vi "frequency_response.vi"() -> ()   [LabVIEW 2012]
uses:
  Trace controls.ctl
  probe_point.ctl
  injection_point.ctl
  pose_selector.ctl
  pose_source.ctl
  pose_relative_to.ctl
  <vilib>/Platform/TimedLoop/XDataNode/timing_clust.ctl
  <vilib>/Platform/TimedLoop/XDataNode/nitl_modes.ctl
  <vilib>/Platform/TimedLoop/XDataNode/wakeup.ctl
  <vilib>/Utility/error.llb/DialogType.ctl
  <vilib>/Utility/file.llb/Write To Spreadsheet File (string).vi
  initialization/micron_globals.vi
  <vilib>/Platform/TimedLoop/XDataNode/XDataNode.xnode
  <vilib>/Platform/TimedLoop/XDataNode/XDNodeRunTimeDep.lvlib
  <vilib>/Analysis/NI_AALPro.lvlib
  <vilib>/gmath/NI_Gmath.lvlib
panel:
  in  "Pose response":T1[](array[typedef])
  in  "Use Output Enable":bool=TRUE
  out "Report":string[][](table)
  in  "Report file":path=path "c:/test/freq_reponse.csv"
  in  "Save report":bool
  in  "Store":T4(radio)=enum."Radio Selection 7"
  in  "Graph?":bool[](array[boolean])=[TRUE, TRUE, TRUE, TRUE, TRUE, TRUE, FALSE]
  in  "Name":string[](array[string])
  in  "Delay":sgl=0.0031 format="%#_3p"
  out "Responses":waveform(sgl)[](graph)
  out "Reference":waveform(sgl)[](graph)
  in  "Reference signal":T5[](array[typedef])=[{"+ stim"=TRUE, "Relative"=FALSE, "Scale"=enum."1X", "Probe point"=enum."Output 0", "XYZ selector"={"Boolean"=TRUE, "Boolean 2"=FALSE, "Boolean 3"=FALSE}, "To tip"=FALSE}, {"+ stim"=FALSE, "Relative"=FALSE, "Scale"=enum."1X", "Probe point"=enum."Position (tip)", "XYZ selector"={"Boolean"=FALSE, "Boolean 2"=FALSE, "Boolean 3"=FALSE}, "To tip"=FALSE}, {"+ stim"=FALSE, "Relative"=FALSE, "Scale"=enum."1X", "Probe point"=enum."Position (tip)", "XYZ selector"={"Boolean"=FALSE, "Boolean 2"=FALSE, "Boolean 3"=FALSE}, "To tip"=FALSE}, {"+ stim"=FALSE, "Relative"=FALSE, "Scale"=enum."1X", "Probe point"=enum."Position (tip)", "XYZ selector"={"Boolean"=FALSE, "Boolean 2"=FALSE, "Boolean 3"=FALSE}, "To tip"=FALSE}]
  out "Driven axis":i32
  in  "Scanning":bool
  in  "Scan":bool
  in  "Stimulus":T8={"Injection point"=enum."Output", "Closed loop"=TRUE, "Tip -> world"=FALSE, "Amplitude"=10.0, "Type"=enum."Arbitrary", "Phase"=0.0, "Frequency"=0.0, "Length"=0.0} {"Length" min=0.0 max=100.0 step=100.0 format="%#_4p"; "Frequency" min=0.0 step=100.0 format="%#_4g"; "Phase" min=-180.0 max=360.0 step=100.0 format="%#.2f"; "Amplitude" format="%#_3p"}
  in  "Scan axes":bool[](array[boolean])=[TRUE, TRUE, TRUE, TRUE, TRUE, TRUE]
  in  "Max off-axis":bool=TRUE
  in  "Integrator scaling":bool=TRUE
  in  "Frequency range":cluster{"Min":dbl, "Max":dbl}={"Min"=10.0, "Max"=250.0} {"Max" format="%#_3p"; "Min" format="%#_3p"}
  in  "N points":u32=30
  in  "Window":T9(ring)
  in  "Restart Averaging":bool
  in  "Unwrap phase":bool
  in  "Averaging Parameters":T10={"averaging mode"=0, "weighting mode"=1, "number of averages"=10} {"averaging mode" items=["No averaging", "Vector averaging", "RMS averaging", "Peak hold"]; "weighting mode" items=["Linear", "Exponential"]}
  in  "Phase offset":sgl=90.0
  out "Status":string
  out "Phase":T11(graph)
  out "Amplitude":cluster{"X":dbl[], "Y":dbl[]}[](graph)
  in  "Response signals":T5[](array[typedef])=[{"+ stim"=FALSE, "Relative"=FALSE, "Scale"=enum."1X", "Probe point"=enum."Link pos 0", "XYZ selector"={"Boolean"=TRUE, "Boolean 2"=TRUE, "Boolean 3"=TRUE}, "To tip"=FALSE}, {"+ stim"=FALSE, "Relative"=FALSE, "Scale"=enum."1X", "Probe point"=enum."Link pos 1", "XYZ selector"={"Boolean"=TRUE, "Boolean 2"=TRUE, "Boolean 3"=TRUE}, "To tip"=FALSE}, {"+ stim"=FALSE, "Relative"=FALSE, "Scale"=enum."1X", "Probe point"=enum."Position (tip)", "XYZ selector"={"Boolean"=FALSE, "Boolean 2"=FALSE, "Boolean 3"=FALSE}, "To tip"=FALSE}, {"+ stim"=FALSE, "Relative"=FALSE, "Scale"=enum."1X", "Probe point"=enum."Position (tip)", "XYZ selector"={"Boolean"=FALSE, "Boolean 2"=FALSE, "Boolean 3"=FALSE}, "To tip"=FALSE}]
  # "Result buffers"
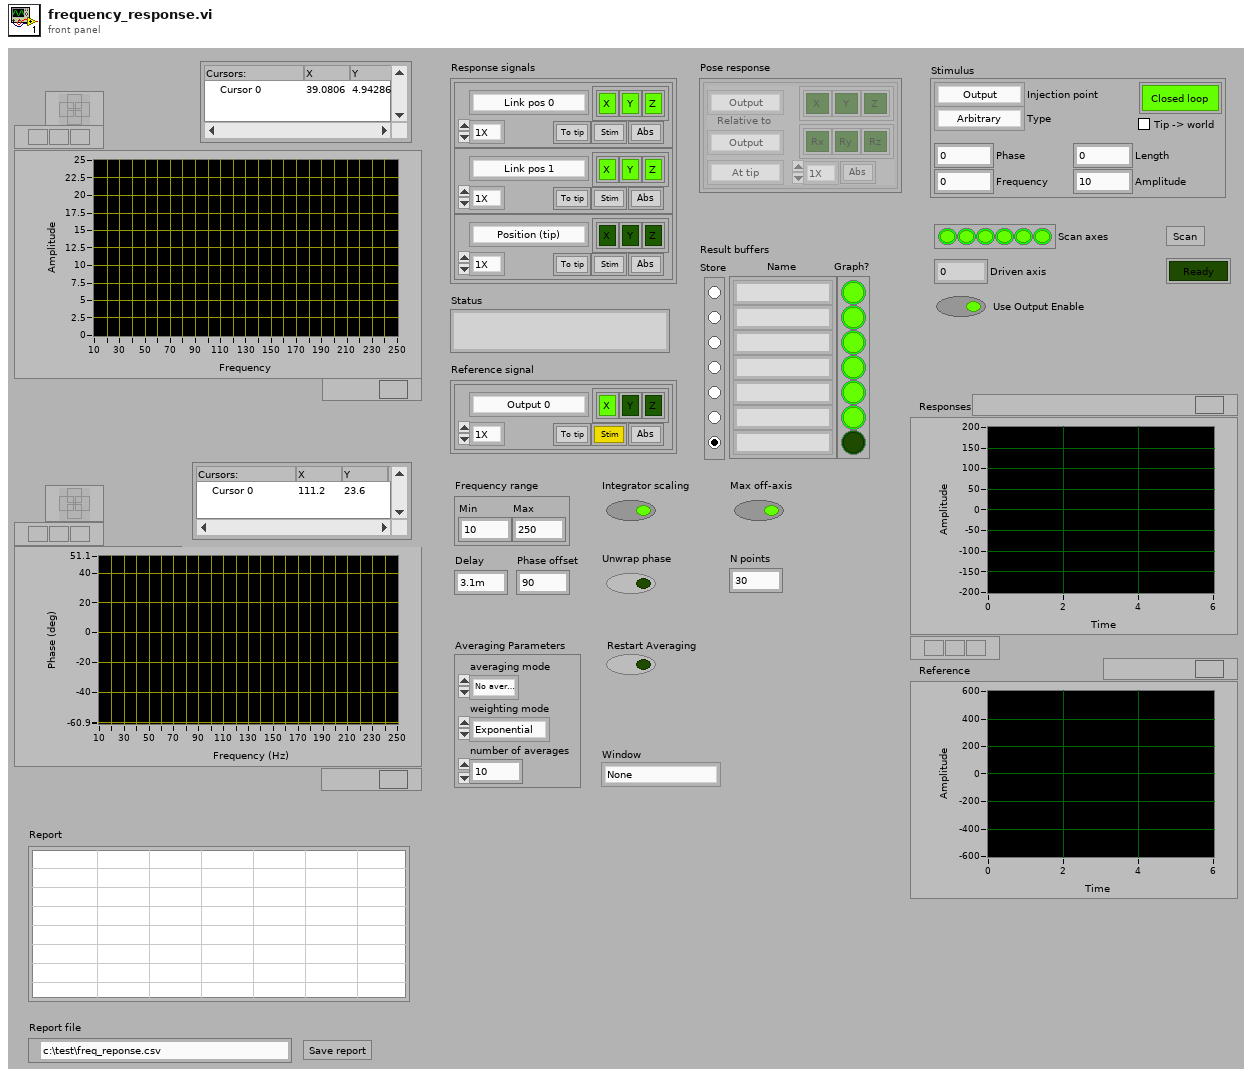
[diagram p1: front panel]
types:
  T1 = typedef "pose_selector.ctl" = cluster{"Scale":enum16{"1X", "10X", "100X", "1KX", "10KX"}, "Source":T2, "XYZ selector":cluster{"Boolean":bool, "Boolean 2":bool, "Boolean 3":bool}, "RPY selector":cluster{"Boolean":bool, "Boolean 2":bool, "Boolean 3":bool}, "Relative to":T3, "Relative":bool, "Translate":enum16{"At tip", "At RCM", "At KC", "At origin"}}
  T2 = typedef "pose_source.ctl" = enum16{"Output", "Handle", "Handle KF", "Goal", "Absolute"}
  T3 = typedef "pose_relative_to.ctl" = enum16{"Output", "Handle", "Handle KF", "Goal", "Absolute", "Trace start"}
  T4 = enum32{"Radio Selection 1", "Radio Selection 2", "Radio Selection 3", "Radio Selection 4", "Radio Selection 5", "Radio Selection 6", "Radio Selection 7"}
  T5 = typedef "Trace controls.ctl" = cluster{"+ stim":bool, "Relative":bool, "Scale":enum16{"1X", "10X", "100X", "1KX", "10KX"}, "Probe point":T6, "XYZ selector":cluster{"Boolean":bool, "Boolean 2":bool, "Boolean 3":bool}, "To tip":bool}
  T6 = typedef "probe_point.ctl" = enum16{"Position (tip)", "Position (RCM)", "Null pos (tip)", "Null pos (RCM)", "V limiter (tip)", "V Limiter (RCM)", "Goal (tip)", "Goal (RCM)", "Link pos 0", "Link pos 1", "KF link pos 0", "KF link pos 1", "Link rate 0", "Link rate 1", "Link residue 0", "Link residue 1", "Link goal 0", "Link goal 1", "Rate limit 0", "Rate limit 1", "Link error 0", "Link error 1", "Controller 0", "Controller 1", "Output 0", "Output 1", "Drive 0", "Drive 1", "Stimulus 0", "Stimulus 1", "Trace data 0", "Trace data 1", "Analog data 0", "Analog data 1", "Status flags", "Light 0", "Light 1", "Light 2", "Light 3", "Light 4", "Light 5", "Goal origin", "Goal rotation 0", "Goal rotation 1", "Goal rotation 2", "Output origin", "Output rotation 0", "Output rotation 1", "Output rotation 2", "Handle origin", "Handle rotation 0", "Handle rotation 1", "Handle rotation 2", "Handle position", "Handle velocity", "Handle acceleration", "Handle angles", "Handle angle rates", "Handle pos residue", "Handle angle residue", "Trace length"}
  T7 = typedef "injection_point.ctl" = enum16{"Total pose", "V limiter", "Goal ", "Link position", "KF link position", "Inverse kin", "Link goal", "Link error", "Controller", "Output", "Drive", "Light"}
  T8 = cluster{"Injection point":T7, "Closed loop":bool, "Tip -> world":bool, "Amplitude":sgl, "Type":enum16{"Off", "Step", "Sine", "Triangle", "Arbitrary"}, "Phase":dbl, "Frequency":dbl, "Length":dbl}
  T9 = enum16{"None ", "Hanning", "Hamming", "Blackman-Harris", "Exact Blackman", "Blackman", "Flat Top", "4 Term B-Harris ", "7 Term B-Harris", "Low Sidelobe"}
  T10 = cluster{"averaging mode":u16, "weighting mode":u16, "number of averages":u32}
  T11 = cluster{"X out":dbl[], "Unwrapped Phase":dbl[]}[]
  T12 = typedef "XDNodeRunTimeDep.lvlib/timing_clust.ctl" = cluster{"Expected End [f-1]":u64, "Actual End [f-1]":u64, "Finished Late? [f-1]":bool, "Expected End [i-1]":u64, "Actual End [i-1]":u64, "Finished Late? [i-1]":bool, "Expected Start [i]":u64, "Actual Start [i]":u64, "Expected Start [f]":u64, "Actual Start [f]":u64, "Source Name":string, "Structure Name":string, "Period":i64, "Deadline":i64, "Offset":i64, "Start":i64, "Priority":i32, "Timeout":i32, "Mode":T13, "Wakeup Reason":T14, "Error":errorcluster, "Source Type":string, "Secondary Source Type":string, "Global End Time":u64, "Global Start Time":u64, "Frame Duration":u64, "Iteration Duration":u64, "Assigned CPU":i32, "I/O Scan Engine Mode":u32}
  T13 = typedef "XDNodeRunTimeDep.lvlib/nitl_modes.ctl" = enum32{"No Change", "Process missed periods, maintain original phase", "Discard missed periods, maintain original phase", "Process missed periods, ignore original phase", "Discard missed periods, ignore original phase"}
  T14 = typedef "XDNodeRunTimeDep.lvlib/wakeup.ctl" = enum32{"Normal", "Aborted", "Asynchronous wakeup", "Timing source error", "Timed loop error", "Timeout"}
  T15 = cluster{"Averaging Parameters":cluster{"averaging mode":u16, "weighting mode":u16, "number of averages":u32}, "Window":enum16{"None ", "Hanning", "Hamming", "Blackman-Harris", "Exact Blackman", "Blackman", "Flat Top", "4 Term B-Harris ", "7 Term B-Harris", "Low Sidelobe"}, "Reference signal":T5[]}
  T16 = cluster{"Phase offset":sgl, "Unwrap phase ":bool, "N points":u32, "Integrator scaling":bool, "Frequency range":cluster{"Min":dbl, "Max":dbl}, "Max off-axis":bool, "Graph?":bool[], "Name":string[], "Delay":sgl}
  T17 = enum8{"Enabled", "Disabled", "Disabled and Grayed Out"}
  T18 = typedef "DialogType.ctl" = u16
  T19 = enum16{"Off", "Step", "Sine", "Triangle", "Arbitrary"}
  T20 = typedef "Micron params.ctl" = cluster{"Stimulus":T21, "Goal Filter A":T22, "Mode controls":T23, "Manipulator type":enum16{"Current piezo", "Voltage piezo"}, "Manipulator calibration":T24, "Network":T26, "Goal Filter B":T22, "Cancellation":T27, "Transition time":sgl, "Estimation":T29}
  T21 = typedef "stimulus.ctl" = cluster{"Type":enum16{"Off", "Step", "Sine", "Triangle", "Arbitrary"}, "Phase":dbl, "Amplitude":sgl[], "Injection point":T7, "Closed loop":bool, "Offset":sgl[], "Tip -> world":bool, "Frequency":dbl, "Length":dbl}
  T22 = typedef "goal_loop_parms.ctl" = cluster{"Speedup max":sgl, "Speedup thresh":sgl, "Speedup nonlin":sgl, "Filters":cluster{"Lower Fc":sgl, "Lower Q":sgl, "Scale factor":sgl, "Upper Fc":sgl, "Upper Q":sgl, "V limit":sgl, "V limit range":sgl}[]}
  T23 = typedef "mode_conrols.ctl" = cluster{"Hold":bool, "Cancellation":bool, "Goal filter":bool, "Trigger":bool}
  T24 = typedef "manipulator_cal.ctl" = cluster{"Tool offsets":sgl[][], "Tip light calibration":T25, "Handle light calibration":T25, "Base pivots":sgl[][], "Output pivots":sgl[][], "Length center":sgl, "Workspace height":sgl[], "Workspace diameter":sgl[], "Linearization":sgl[][], "Stack travel":sgl, "Saturation pos":sgl, "Inverse filters":cluster{"filter structure":enum32{"IIR 2nd Order", "IIR 4th Order"}, "Reverse Coefficients":dbl[], "Forward Coefficients":dbl[]}[]}
  T25 = typedef "probe_calibration.ctl" = sgl[][]
  T26 = typedef "network_params.ctl" = cluster{"Remote Host":string, "Send Status":bool, "Send Port":u16, "Recv Commands":bool, "Recv Port":u16}
  T27 = typedef "sq_control_params.ctl" = cluster{"KP":T28, "KI":sgl, "KD":T28, "Max vel":sgl, "Max acc":sgl, "Int error limit":sgl, "RCM gain":sgl, "Bypass":bool, "Degraded gain":sgl}
  T28 = typedef "decoupled_gain.ctl" = cluster{"XY":sgl, "Rxy":sgl, "Z":sgl, "Rz":sgl}
  T29 = typedef "estimation_controls.ctl" = cluster{"Link":cluster{"Measure noise":dbl[], "Process noise":dbl[], "Alt process noise":dbl[], "Alt turnoff cycles":i32, "Innovation limit":dbl[], "Residue threshold":dbl, "Enable":bool}, "Handle":cluster{"Measure noise":dbl[], "Process noise":dbl[], "State limits":dbl[], "Innovation limit":dbl[], "Prediction Lookahead":sgl, "Enable":bool}}
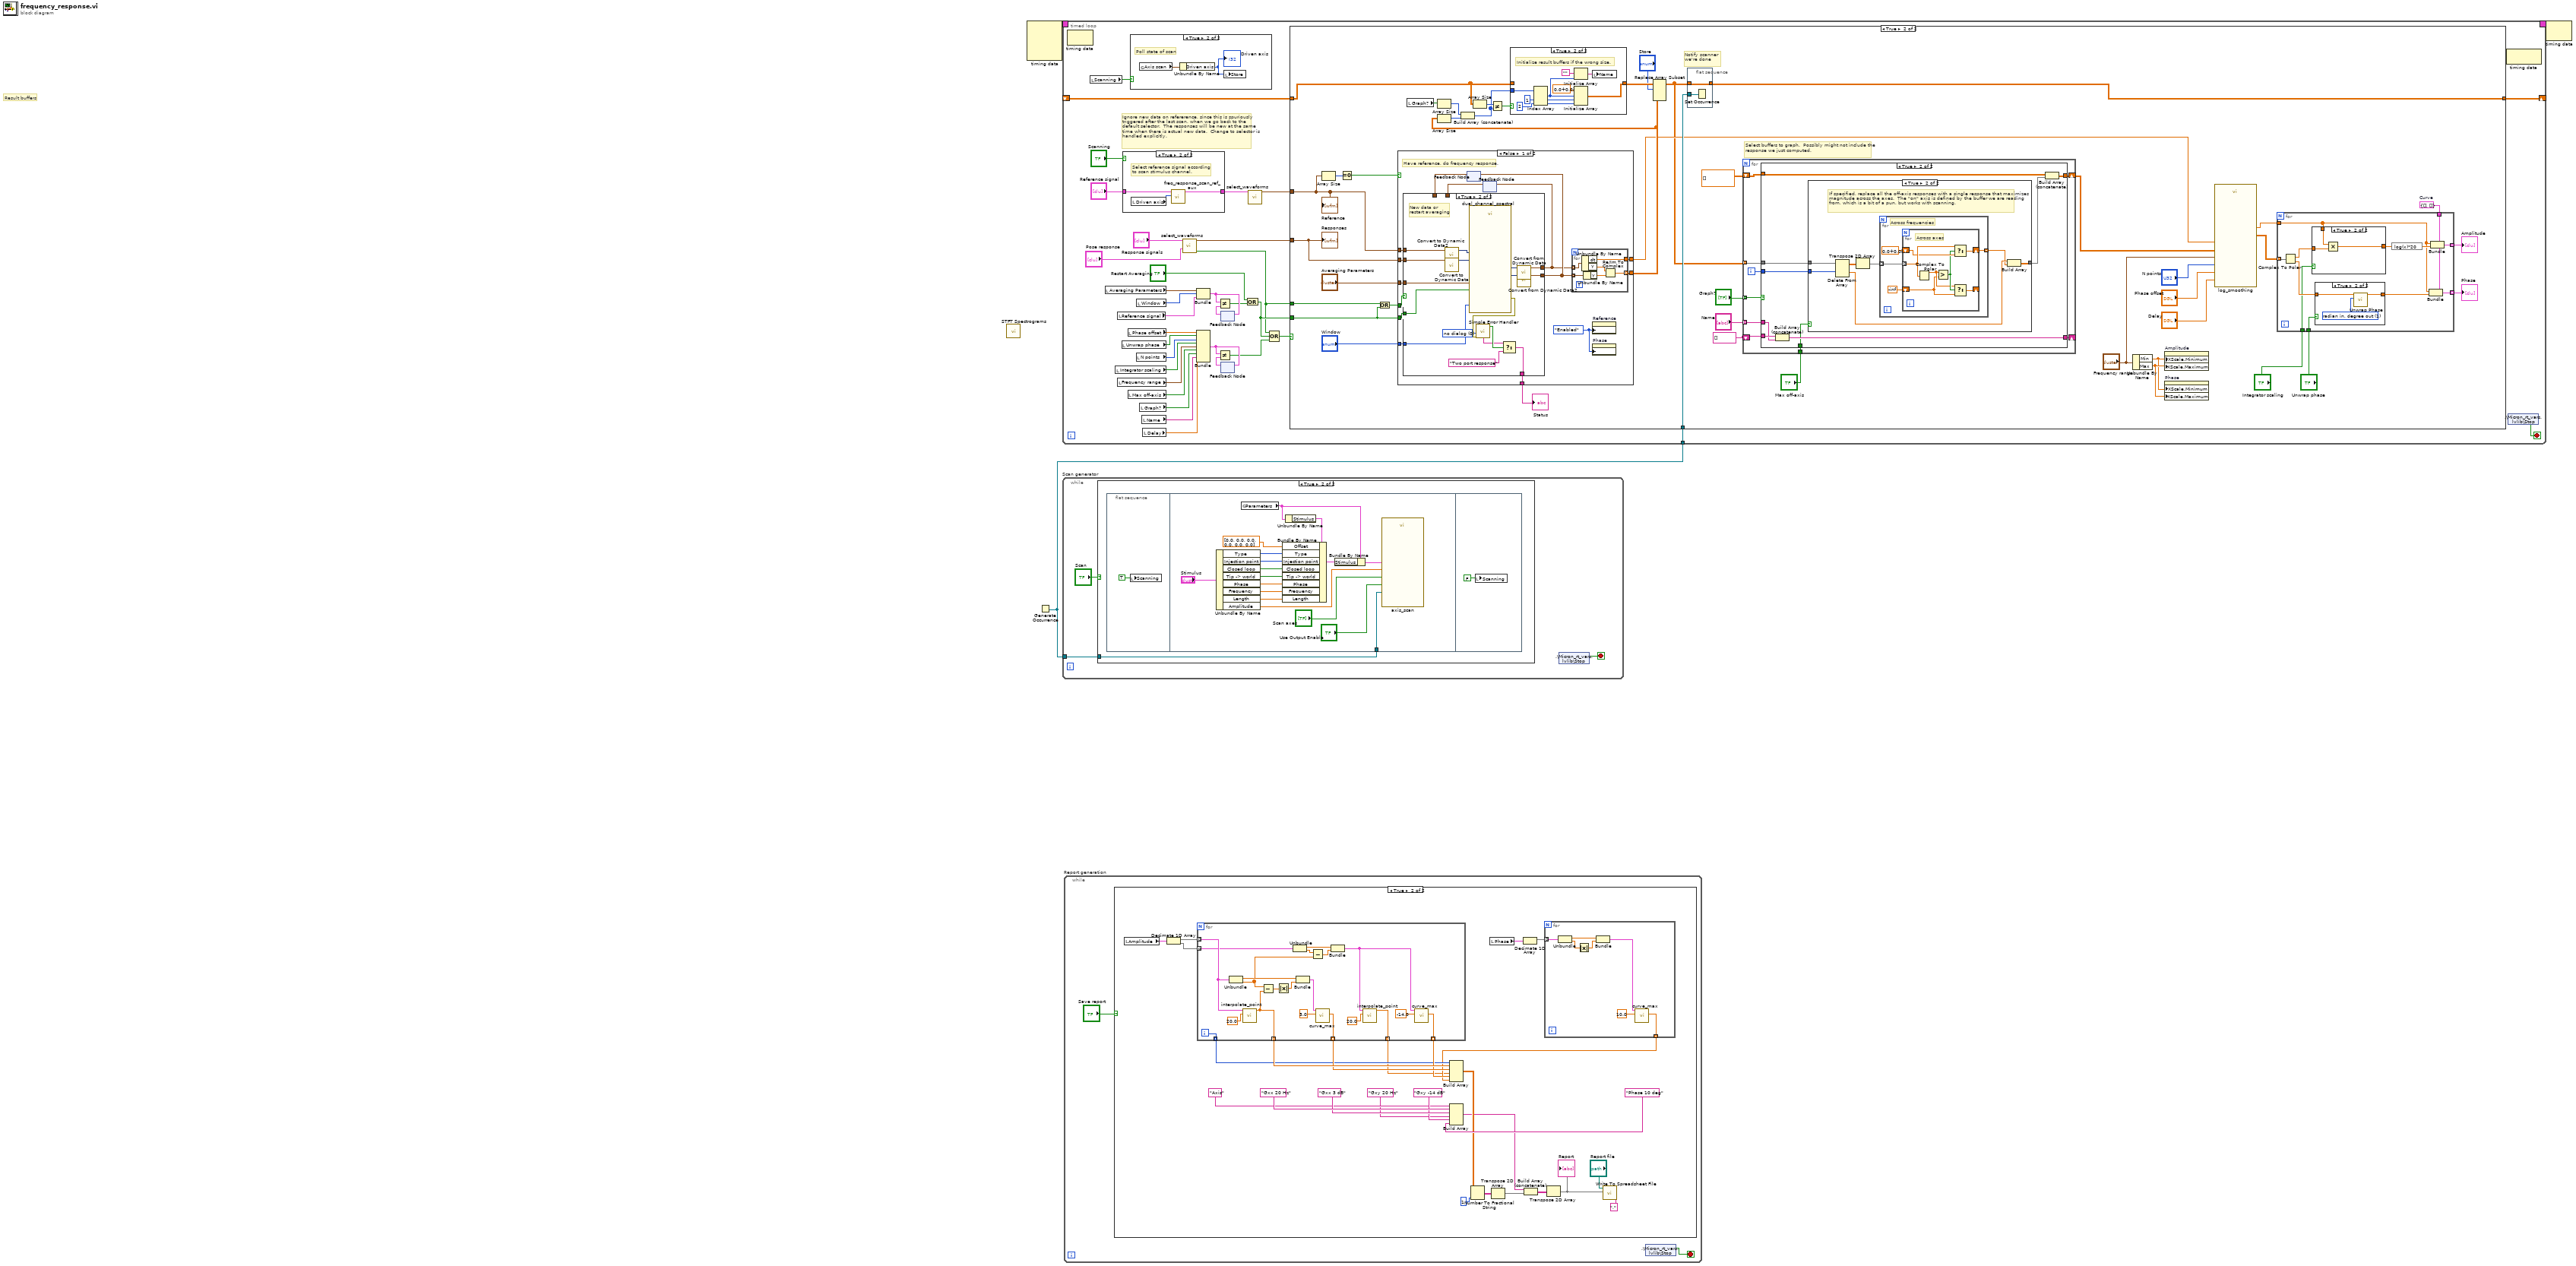
[diagram p0: block diagram]
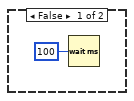
[diagram p2: hidden frame]
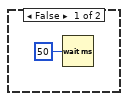
[diagram p3: hidden frame]
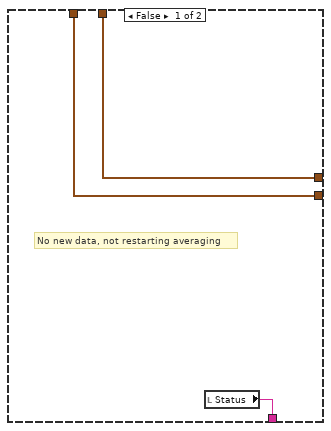
[diagram p7: hidden frame]
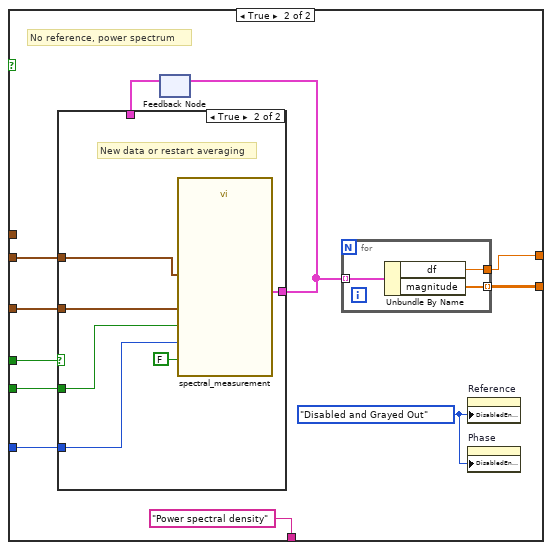
[diagram p8: hidden frame]
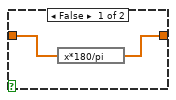
[diagram p14: hidden frame]
diagram:
  # "Result buffers"
  n1 = call <vilib>:"STFT Spectrograms.vi"() -> ()  [unwired: 10 in, 2 out]
  n2 = node-c288() -> (w3:T12)  [unwired: 4 out]
  n3 = Generate Occurrence() -> (w1:refnum<k4>)
  n4 = timed-loop {
    timing: w3 -> [_]
    timing-out: [_] -> w2
    shift-right: [w19] -> _
    shift-left: _ -> [w20]
    tunnel: w1 -> [w15]
    stop <- w8 stop-if-true
    # "Ignore new data on refererence, since this is spuriously triggered after the last scan, when we go back to the default selector.  The responses will be new at the same time when there is actual new data.  Change to selector is handled explicitly."
    n5 = node-c288() -> ()  [unwired: 2 out]
    n6 = local read "Scanning"() -> (w7:bool)
    n7 = local read "Averaging Parameters"() -> (w36:T10)
    n8 = local read "Integrator scaling"() -> (w31:bool)
    n9 = local read "Reference signal"() -> (w6:T5[])
    n10 = local read "Frequency range"() -> (w30:cluster{"Min":dbl, "Max":dbl})
    n11 = local read "Unwrap phase"() -> (w33:bool)
    n12 = case shown="True" "Scanning" {
      tunnel: "Reference signal" -> [w40 w43]
      tunnel: [w40 w42] -> w13
      frame False {
      }
      frame True {
        # "Select reference signal according  to scan stimulus channel."
        n13 = local read "Driven axis"() -> (w41:i32)
        n14 = call "freq_response_scan_ref_aux.vi"("Testing"=w41, "Trace controls in"=w43) -> ("Trace controls out"=w42:T5[])  [unwired: 9 in]
      }
    }
    n15 = local read "Phase offset"() -> (w34:sgl)
    n16 = local read "Max off-axis"() -> (w16:bool)
    n17 = case shown="True" w7 {
      frame False {
      }
      frame True {
        # "Poll state of scan"
        n18 = global read "micron_globals.vi" "Axis scan"() -> (w39:cluster{"Driven axis":i32, "Scan index":i32})
        n19 = Unbundle By Name(w39) -> ("Driven axis"=w38:i32)
        "Driven axis" <- w38
        n20 = local write "Store"(w38) -> ()
      }
    }
    n21 = local read "N points"() -> (w32:u32)
    n22 = local read "Window"() -> (w35:T9)
    n23 = local read "Graph?"() -> (w17:bool[])
    n24 = local read "Name"() -> (w18:string[])
    n25 = local read "Delay"() -> (w10:sgl)
    n26 = call "select_waveforms.vi"("Trace controls"="Response signals", "Pose selectors"="Pose response") -> ("Waveforms out"=w37:waveform(sgl)[], "New data"=w5:bool)  [unwired: 10 in, 2 out]
    n27 = Bundle("Averaging Parameters"=w36, "Window"=w35, "Reference signal"=w6) -> (w26:T15)  [unwired: 1 in]
    n28 = Bundle("Phase offset"=w34, "Unwrap phase"=w33, "N points"=w32, "Integrator scaling"=w31, "Frequency range"=w30, "Max off-axis"=w16, "Graph?"=w17, "Name"=w18, "Delay"=w10) -> (w29:T16)  [unwired: 1 in]
    n29 = feedback #1() -> (w27:T15)  [unwired: 1 in]
    n30 = Not Equal?(x=w26, y=w27) -> (x != y?=w23:bool)
    n31 = feedback-in #1(w26) -> ()
    n32 = feedback-in #2(w29) -> ()
    n33 = feedback #2() -> (w28:T16)  [unwired: 1 in]
    n34 = Not Equal?(x=w29, y=w28) -> (x != y?=w25:bool)
    n35 = Compound Arithmetic op=OR("Restart Averaging", w23) -> (w21:bool)
    n36 = call "select_waveforms.vi"("Trace controls"=w13) -> ("Waveforms out"=w12:waveform(sgl)[])  [unwired: 11 in, 3 out]
    n37 = Compound Arithmetic op=OR(w5, w21, w25) -> (w24:bool)
    n38 = case shown="True" w24 {
      tunnel: w37 -> [_ w46]
      tunnel: w21 -> [_ w80]
      tunnel: w5 -> [_ w79]
      tunnel: w20 -> [w44 w78]
      tunnel: [w44 w76] -> w19
      tunnel: w15 -> [_ w72]
      tunnel: w12 -> [_ w87]
      frame False {
      }
      frame True {
        w47 = cluster{"X":dbl[], "Y":dbl[]} {"X"=[], "Y"=[]}  # Curve
        # "Select buffers to graph.  Possibly might not include the response we just computed."
        # "Notify scanner we're done"
        n39 = Array Size(array=w87) -> (size(s)=w71:i32)
        n40 = Equal To 0?(x=w71) -> (x = 0?=w45:bool)
        n41 = Or(x=w79, y=w80) -> (x .or. y?=w64:bool)
        n42 = case shown="False" w45 {
          tunnel: [w101 "Power spectral density" ("message")] -> w85
          tunnel: "Averaging Parameters" -> [w100 w133]
          tunnel: "Window" -> [w99 w134]
          tunnel: w80 -> [w98 w135]
          tunnel: [w97 w131] -> w65
          tunnel: w64 -> [w92 w136]
          tunnel: [w91 w130] -> w86
          tunnel: w87 -> [w90 _]
          tunnel: w46 -> [w89 w132]
          frame False {
            w88 = T17."Enabled" ("Disabled")
            # "Have reference, do frequency response."
            n43 = feedback #3() -> (w93:waveform(dbl)[])  [unwired: 1 in]
            n44 = feedback #4() -> (w94:waveform(dbl)[])  [unwired: 1 in]
            n45 = case shown="True" w92 {
              tunnel: w89 -> [_ w106]
              tunnel: w98 -> [_ w115]
              tunnel: w100 -> [_ w114]
              tunnel: w99 -> [_ w113]
              tunnel: [w104 w110] -> w95
              tunnel: [w103 w109] -> w96
              tunnel: w94 -> [w104 _]
              tunnel: w93 -> [w103 _]
              tunnel: [w102 w116] -> w101
              tunnel: w90 -> [_ w107]
              frame False {
                # "No new data, not restarting averaging"
                n46 = local read "Status"() -> (w102:string)
              }
              frame True {
                w105 = T18 0 items=["no dialog", "OK message", "continue or stop message", "OK message + warnings", "continue/stop + warnings"] ("type of dialog (OK msg:1)")
                # "New data or\nrestart averaging"
                n47 = call "Convert to Dynamic Data2"("Array of Waveforms"=w107) -> ("Dynamic Data Type"=w108:dynamicdata)  [unwired: 3 out]
                n48 = call "Convert to Dynamic Data"("Array of Waveforms"=w106) -> ("Dynamic Data Type"=w121:dynamicdata)  [unwired: 3 out]
                n49 = call "dual_channel_spectral.vi"("Input Signal A"=w108, "Input Signal B"=w121, "Restart Averaging (F)"=w115, "Averaging parameters"=w114, "Window"=w113) -> ("Imaginary"=w111:dynamicdata, "Real"=w112:dynamicdata, "error out"=w120:errorcluster)  [unwired: 9 in, 3 out]
                n50 = call <vilib>:"Simple Error Handler.vi"("type of dialog (OK msg:1)"=w105, "error in (no error)"=w120) -> ("error?"=w119:bool, "message"=w118:string)  [unwired: 6 out]
                n51 = Select(t=w118, s=w119, f="Two port response") -> (s? t:f=w116:string)
                n52 = call "Convert from Dynamic Data"("Dynamic Data Type"=w112) -> ("Array of Waveform"=w110:waveform(dbl)[])  [unwired: 3 in]
                n53 = call "Convert from Dynamic Data2"("Dynamic Data Type"=w111) -> ("Array of Waveform"=w109:waveform(dbl)[])  [unwired: 3 in]
              }
            }
            n54 = feedback-in #3(w96) -> ()
            n55 = feedback-in #4(w95) -> ()
            n56 = for {
              tunnel: w95 -> [w125] mode=indexing
              tunnel: w96 -> [w126] mode=indexing
              tunnel: [w124] -> w91 mode=indexing
              tunnel: [w122] -> w97
              n57 = Unbundle By Name(w125) -> ("dt"=w122:dbl, "Y"=w123:dbl[])
              n58 = Unbundle By Name(w126) -> ("Y"=w127:dbl[])
              n59 = Re/Im To Complex(1:w127, 2:w123) -> (0:w124:cdb[])
            }
            n60 = property on="Reference" class="WFGraph (strict)"("DisabledEnum"=w88) -> ()  [unwired: 2 in, 2 out]
            n61 = property on="Phase" class="XYGraph (strict)"("DisabledEnum"=w88) -> ()  [unwired: 2 in, 2 out]
          }
          frame True {
            w128 = T17."Disabled and Grayed Out" ("Disabled")
            # "No reference, power spectrum"
            n62 = feedback #5() -> (w138:cluster{"f0":dbl, "df":dbl, "magnitude":dbl[]}[])  [unwired: 1 in]
            n63 = case shown="True" w136 {
              tunnel: [w142 w148] -> w137
              tunnel: w138 -> [w142 _]
              tunnel: w135 -> [_ w146]
              tunnel: w134 -> [_ w145]
              tunnel: w133 -> [_ w144]
              tunnel: w132 -> [_ w143]
              frame False {
                # "No new data, not\nrestarting averaging"
              }
              frame True {
                # "New data or restart averaging"
                n64 = call "spectral_measurement.vi"("Signals"=w143, "Restart Averaging"=w146, "dB On"=FALSE, "Spectrum Averaging Parameters"=w144, "Window"=w145) -> ("PSD"=w148:cluster{"f0":dbl, "df":dbl, "magnitude":dbl[]}[])  [unwired: 8 in, 2 out]
              }
            }
            n65 = feedback-in #5(w137) -> ()
            n66 = for {
              tunnel: w137 -> [w141] mode=indexing
              tunnel: [w140] -> w131
              tunnel: [w139] -> w130 mode=indexing
              n67 = Unbundle By Name(w141) -> ("df"=w140:dbl, "magnitude"=w139:dbl[])
            }
            n68 = property on="Reference" class="WFGraph (strict)"("DisabledEnum"=w128) -> ()  [unwired: 2 in, 2 out]
            n69 = property on="Phase" class="XYGraph (strict)"("DisabledEnum"=w128) -> ()  [unwired: 2 in, 2 out]
          }
        }
        "Status" <- w85
        n70 = local read "Graph?"() -> (w59:bool[])
        n71 = Array Size(array=w59) -> (size(s)=w58:i32)
        n72 = Array Size(array=w86) -> (size(s)=w63:i32[])
        n73 = Build Array (concatenate)(w58, w63) -> (w60:i32[])
        n74 = Array Size(array=w78) -> (size(s)=w62:i32[])
        n75 = Not Equal?(x=w62, y=w60) -> (x != y?=w61:bool)
        n76 = case shown="True" w61 {
          tunnel: w78 -> [w190 _]
          tunnel: w60 -> [_ w199]
          tunnel: [w190 w194] -> w57
          frame False {
          }
          frame True {
            # "Initialize result buffers if the wrong size."
            n77 = Index Array(array=w199, index #2=1 ("index"), index #3=2 ("index")) -> (element #1=w192:i32, element #2=w196:i32, element #3=w195:i32)  [unwired: 1 in]
            n78 = Initialize Array("", w192) -> (w191:string[])
            n79 = Initialize Array(cdb 0.0+0.0i, w192, w196, w195) -> (w194:cdb[][][])
            n80 = local write "Name"(w191) -> ()
          }
        }
        n81 = Replace Array Subset(array=w57, new element=w86, index (dim 0)="Store") -> (w51:cdb[][][])  [unwired: 2 in]
        n82 = flat-sequence {
          tunnel: w51 -> [w150]
          tunnel: [w150] -> w76
          tunnel: w72 -> [w149]
          frame #0 {
            n83 = Set Occurrence(w149) -> ()
          }
        }
        n84 = for {
          tunnel: "Graph?" -> [w159] mode=indexing
          tunnel: w51 -> [w157] mode=indexing
          shift-right: [w156] -> w50
          shift-left: cdb[][] [] -> [w158]
          tunnel: "Name" -> [w153] mode=indexing
          shift-right: [w155] -> _
          shift-left: string[] [] ("Name") -> [w154]
          tunnel: "Max off-axis" -> [w152]
          i -> [w151]
          n85 = case shown="True" w159 {
            tunnel: w158 -> [w161 w170]
            tunnel: w157 -> [_ w165]
            tunnel: [w161 w169] -> w156
            tunnel: [w160 w168] -> w155
            tunnel: w154 -> [w160 w167]
            tunnel: w153 -> [_ w166]
            tunnel: w152 -> [_ w164]
            tunnel: w151 -> [_ w162]
            frame False {
            }
            frame True {
              n86 = Build Array (concatenate)(w167, w166) -> (w168:string[])
              n87 = case shown="True" w164 {
                tunnel: w165 -> [w171 w178]
                tunnel: [w171 w173] -> w163
                tunnel: w162 -> [_ w172]
                frame False {
                }
                frame True {
                  # "If specified, replace all the off-axis responses with a single response that maximizes magnitude across the axes.  The \"on\" axis is defined by the buffer we are reading from, which is a bit of a pun, but works with scanning."
                  n88 = Delete From Array(array=w178, index (row)=w172) -> (deleted portion=w175:cdb[], array with subset deleted=w177:cdb[][])  [unwired: 2 in]
                  n89 = Transpose 2D Array(2D array=w177) -> (transposed array=w176:cdb[][])
                  n90 = for {
                    tunnel: w176 -> [w182] mode=indexing
                    tunnel: [w179] -> w174 mode=indexing
                    # "Across frequencies"
                    n91 = for {
                      tunnel: w182 -> [w188] mode=indexing
                      shift-right: [w186] -> _
                      shift-left: -inf -> [w183]
                      shift-right: [w189] -> w179
                      shift-left: cdb 0.0+0.0i -> [w187]
                      # "Across axes"
                      n92 = Complex To Polar(r * e^(i*theta)=w188) -> (r=w184:dbl)  [unwired: 1 out]
                      n93 = Greater?(x=w184, y=w183) -> (0:w185:bool)
                      n94 = Select(t=w188, s=w185, f=w187) -> (s? t:f=w189:cdb)
                      n95 = Select(t=w184, s=w185, f=w183) -> (s? t:f=w186:dbl)
                    }
                  }
                  n96 = Build Array(w175, w174) -> (w173:cdb[][])
                }
              }
              n97 = Build Array (concatenate)(w170, w163) -> (w169:cdb[][])
            }
          }
        }
        n98 = Unbundle By Name("Frequency range") -> ("Min"=w74:dbl, "Max"=w75:dbl)
        n99 = property on="Amplitude" class="XYGraph (strict)"("XScale.Minimum"=w74, "XScale.Maximum"=w75) -> ()  [unwired: 2 in, 2 out]
        n100 = property on="Phase" class="XYGraph (strict)"("XScale.Minimum"=w74, "XScale.Maximum"=w75) -> ()  [unwired: 2 in, 2 out]
        n101 = call "log_smoothing.vi"("Delay (sec)"="Delay", "N points"="N points", "Phase offset (deg)"="Phase offset", "Y"=w50, "Frequency range"="Frequency range", "Frequency resolution (Hz)"=w65) -> ("Y out"=w69:cdb[][], "X out"=w68:dbl[])  [unwired: 4 in]
        n102 = for {
          tunnel: w69 -> [w212] mode=indexing
          tunnel: w68 -> [w202]
          tunnel: [w211] -> w67 mode=indexing
          tunnel: "Unwrap phase" -> [w210]
          tunnel: [w208] -> w66 mode=indexing
          tunnel: "Integrator scaling" -> [w203]
          tunnel: w47 -> [w201]
          n103 = Complex To Polar(r * e^(i*theta)=w212) -> (r=w204:dbl[], theta=w206:dbl[])
          n104 = case shown="True" w203 {
            tunnel: [w213 w214] -> w205
            tunnel: w204 -> [w213 w216]
            tunnel: w202 -> [_ w215]
            frame False {
            }
            frame True {
              n105 = Multiply(x=w215, y=w216) -> (x*y=w214:dbl[])
            }
          }
          n106 = case shown="True" w210 {
            tunnel: w206 -> [w218 w221]
            tunnel: [w217 w219] -> w209
            frame False {
              n107 = expression code="x*180/pi"(w218) -> (w217:dbl[])
            }
            frame True {
              w220 = 1 items=["radian in, radian out", "radian in, degree out", "degree in, degree out", "degree in, radian out"] ("phase unit")
              n108 = call <vilib>:"Unwrap Phase.vi"("phase unit"=w220, "Phase"=w221) -> ("Unwrapped Phase"=w219:dbl[])  [unwired: 8 in, 1 out]
            }
          }
          n109 = expression code="log(x)*20"(w205) -> (w207:dbl[])
          n110 = Bundle(cluster=w201, "X"=w202, "Y"=w209) -> (w208:cluster{"X":dbl[], "Y":dbl[]})
          n111 = Bundle(cluster=w201, "X"=w202, "Y"=w207) -> (w211:cluster{"X":dbl[], "Y":dbl[]})
        }
        "Phase" <- w66
        "Amplitude" <- w67
        "Responses" <- w46
        "Reference" <- w87
      }
    }
    n112 = node-c288() -> ()  [unwired: 2 out]
    n113 = shared-variable ".\\Micron_rt_vars.lvlib\\Stop"() -> (w8:bool)  [unwired: 2 out]
  }
  n114 = while "Scan generator" {
    tunnel: w1 -> [w225]
    stop <- w224 stop-if-true
    n115 = case shown="True" "Scan" {
      tunnel: w225 -> [_ w228]
      frame False {
        n116 = Wait (ms)(milliseconds to wait=u32 50) -> ()  [unwired: 1 out]
      }
      frame True {
        n117 = flat-sequence {
          tunnel: w228 -> [w235]
          frame #0 {
            n118 = local write "Scanning"(TRUE ("Scanning")) -> ()
          }
          frame #1 {
            n119 = Unbundle By Name("Stimulus") -> ("Type"=w234:T19, "Injection point"=w244:T7, "Closed loop"=w245:bool, "Tip -> world"=w246:bool, "Phase"=w233:dbl, "Frequency"=w232:dbl, "Length"=w231:dbl, "Amplitude"=w237:sgl)
            n120 = global read "micron_globals.vi" "Parameters"() -> (w241:T20)
            n121 = Unbundle By Name(w241) -> ("Stimulus"=w242:T21)
            n122 = Bundle By Name(cluster=w242, "Offset"=sgl[] [0.0, 0.0, 0.0, 0.0, 0.0, 0.0], "Type"=w234, "Injection point"=w244, "Closed loop"=w245, "Tip -> world"=w246, "Phase"=w233, "Frequency"=w232, "Length"=w231) -> (w243:T21)
            n123 = Bundle By Name(cluster=w241, "Stimulus"=w243) -> (w239:T20)
            n124 = call "axis_scan.vi"("Parameters in"=w239, "Next scan occurrence"=w235, "Use Output Enable"="Use Output Enable", "Amplitude"=w237, "Scan axes"="Scan axes") -> ()  [unwired: 6 in, 1 out]
          }
          frame #2 {
            n125 = local write "Scanning"(FALSE ("Scanning")) -> ()
          }
        }
      }
    }
    n126 = shared-variable ".\\Micron_rt_vars.lvlib\\Stop"() -> (w224:bool)  [unwired: 2 out]
  }
  n127 = while "Report generation" {
    stop <- w249 stop-if-true
    n128 = case shown="True" "Save report" {
      frame False {
        n129 = Wait (ms)(milliseconds to wait=u32 100) -> ()  [unwired: 1 out]
      }
      frame True {
        n130 = local read "Amplitude"() -> (w255:cluster{"X":dbl[], "Y":dbl[]}[])
        n131 = Decimate 1D Array(w255) -> (w254:cluster{"X":dbl[], "Y":dbl[]}[], w253:cluster{"X":dbl[], "Y":dbl[]}[])
        n132 = for {
          tunnel: w254 -> [w295] mode=indexing
          tunnel: [w293] -> w276 mode=indexing
          tunnel: [w288] -> w275 mode=indexing
          tunnel: w253 -> [w286] mode=indexing
          tunnel: [w281] -> w274 mode=indexing
          tunnel: [w280] -> w270 mode=indexing
          tunnel: [w277] -> w259 mode=indexing
          i -> [w280]
          n133 = Unbundle(w295) -> ("X"=w294:dbl[], "Y"=w285:dbl[])
          n134 = call "interpolate_point.vi"("x"=sgl 20.0 ("single precision float"), "Curve"=w295) -> ("y"=w293:sgl)  [unwired: 9 in]
          n135 = Subtract(x=w285, y=w293) -> (x-y=w290:dbl[])
          n136 = Absolute Value(x=w290) -> (abs(x)=w289:dbl[])
          n137 = Unbundle(w286) -> ("X"=w282:dbl[], "Y"=w284:dbl[])
          n138 = Bundle("X"=w294, w289) -> (w291:cluster{"X":dbl[], dbl[]})  [unwired: 1 in]
          n139 = Subtract(x=w284, y=w285) -> (x-y=w283:dbl[])
          n140 = call "curve_max.vi"("Ymax"=sgl 3.0 ("single precision float"), "Curve in"=w291) -> ("Xc"=w288:sgl)  [unwired: 9 in]
          n141 = Bundle("X"=w282, w283) -> (w279:cluster{"X":dbl[], dbl[]})  [unwired: 1 in]
          n142 = call "interpolate_point.vi"("x"=sgl 20.0 ("single precision float"), "Curve"=w279) -> ("y"=w277:sgl)  [unwired: 9 in]
          n143 = call "curve_max.vi"("Ymax"=sgl -14.0 ("single precision float"), "Curve in"=w279) -> ("Xc"=w281:sgl)  [unwired: 9 in]
        }
        n144 = Build Array("Axis", "Gxx 20 Hz", "Gxx 3 dB", "Gxy 20 Hz", "Gxy -14 dB", "Phase 10 deg") -> (w264:string[])
        n145 = local read "Phase"() -> (w257:T11)
        n146 = Decimate 1D Array(w257) -> (w256:T11)  [unwired: 1 out]
        n147 = for {
          tunnel: w256 -> [w300] mode=indexing
          tunnel: [w297] -> w268 mode=indexing
          n148 = Unbundle(w300) -> ("X out"=w301:dbl[], "Unwrapped Phase"=w299:dbl[])
          n149 = Absolute Value(x=w299) -> (abs(x)=w302:dbl[])
          n150 = Bundle("X out"=w301, w302) -> (w298:cluster{"X out":dbl[], dbl[]})  [unwired: 1 in]
          n151 = call "curve_max.vi"("Ymax"=sgl 10.0 ("single precision float"), "Curve in"=w298) -> ("Xc"=w297:sgl)  [unwired: 9 in]
        }
        n152 = Build Array(w270, w276, w275, w259, w274, w268) -> (w266:sgl[][])
        n153 = Number To Fractional String(number=w266, precision (6)=i16 1) -> (F-format string=w261:string[][])  [unwired: 2 in]
        n154 = Transpose 2D Array(2D array=w261) -> (transposed array=w260:string[][])
        n155 = Build Array (concatenate)(w264, w260) -> (w263:string[][])
        n156 = Transpose 2D Array(2D array=w263) -> (transposed array=w262:string[][])
        "Report" <- w262
        n157 = call-poly <vilib>:"Write To Spreadsheet File.vi"("delimiter (\\t)"="," ("delimiter (\\t)"), "2D data"=w262, "file path (dialog if empty)"="Report file") -> ()  [unwired: 5 in, 1 out]
      }
    }
    n158 = shared-variable ".\\Micron_rt_vars.lvlib\\Stop"() -> (w249:bool)  [unwired: 2 out]
  }
  n159 = node-c288(w2) -> ()  [unwired: 1 out]
